vi "Gripper Controller.vi"(8 "error in":errorcluster) -> ()   [LabVIEW 2017]
doc: "This VI executes continuously carrying out the current operation and responding to updates or new operations. It will often contain the timing or control code that is difficult to place directly in TeleOp. This VI generally opens all sensors and motors and isolates the rest of the robot code from knowing how the operations are carried out."
uses:
  <vilib>/Rock Robotics/WPI/Framework/Completion Status.ctl
  Gripper Setpoints.ctl
  Gripper Operations.ctl
  <vilib>/Rock Robotics/SystemInterfaces/DIO/FPGA_DIOPWMChannel.ctl
  <vilib>/Rock Robotics/WPI/Solenoid/WPI_SolenoidChannel.ctl
  <vilib>/Rock Robotics/WPI/Solenoid/WPI_SolenoidValue.ctl
  <vilib>/Rock Robotics/WPI/MotorControl/WPI_MotorControlOpen SPARK.vi
  <vilib>/Rock Robotics/WPI/Solenoid/WPI_SolenoidOpenDouble.vi
  <vilib>/Rock Robotics/WPI/Solenoid/WPI_SolenoidSetEnum.vi
  <vilib>/addons/control/pid/pid.llb/PID Output Rate Limiter (DBL).vi
  <vilib>/Rock Robotics/SystemInterfaces/AI/FPGA_AIChannel.ctl
  <vilib>/addons/control/pid/NI_PID_pid.lvlib
  <vilib>/ptbypt/NI_PtbyPt.lvlib
panel:
  out "Peak":dbl
  in  "Speed Diff":dbl=0.8 format="%#_13g"
  in  "Peak Current":dbl=80.0
  in  "filter length":i32=50
  in  "output rate":dbl=1000.0 format="%.2f"
  out "Spinning?":bool
  out "Gripper":string
  out "Intake":string
  out "Currents":T1(graph)
  in  "Interactive Values":T2
  out "Current\nCmd":string
  in  "Buttons":cluster{"Execute Cmd":bool, "Abort Cmd":bool}
  out "Command Timing":cluster{"Start Time (ms)":u32, "Iterations":i32}
  out "Status":T4
  # "Interactive Command: You may fill in the settings for a command\nand schedule it with the Execute button. You can observe and abort\nany command while fine tuning the code for the controller."
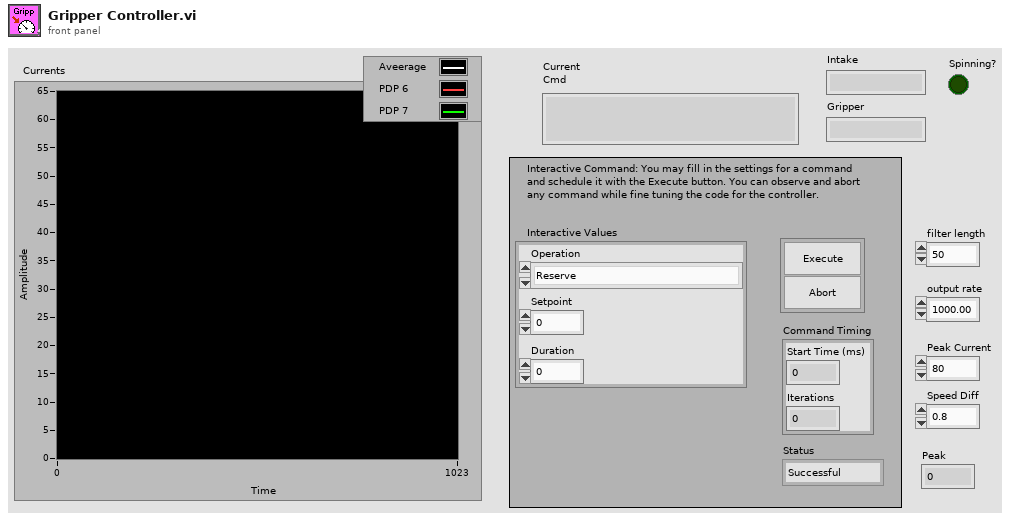
[diagram p1: front panel]
types:
  T1 = cluster{"mean":dbl, "Channel Current":dbl, "Channel Current":dbl}
  T2 = typedef "Gripper Setpoints.ctl" = cluster{"Operation":T3, "Setpoint":dbl, "Duration":dbl}
  T3 = typedef "Gripper Operations.ctl" = enum16{"Reserve", "Read Current", "Immediate", "Open", "Close", "Intake", "Shoot", "Stop"}
  T4 = typedef "Completion Status.ctl" = enum16{"Successful", "Aborted", "Incomplete"}
  T5 = typedef "WPI_SolenoidValue.ctl" = enum16{"Off", "On", "Forward", "Reverse"}
  T6 = typedef "WPI_SolenoidChannel.ctl" = enum8{"Solenoid 0", "Solenoid 1", "Solenoid 2", "Solenoid 3", "Solenoid 4", "Solenoid 5", "Solenoid 6", "Solenoid 7", "Invalid"}
  T7 = typedef "FPGA_DIOPWMChannel.ctl" = enum8{"PWM 0", "PWM 1", "PWM 2", "PWM 3", "PWM 4", "PWM 5", "PWM 6", "PWM 7", "PWM 8", "PWM 9", "PWM MXP 0", "PWM MXP 1", "PWM MXP 2", "PWM MXP 3", "PWM MXP 4", "PWM MXP 5", "PWM MXP 6", "PWM MXP 7", "PWM MXP 8", "PWM MXP 9", "Invalid"}
  T8 = typedef "WPI_SolenoidDevRef.ctl" = cluster{"DevStatus":errorcluster, "Pneumatics Control Module":u8, "Forward Solenoid Channel":T6, "Reverse Solenoid Channel":T6}
  T9 = typedef "WPI_MotorControlDeviceRef.ctl" = cluster{"DeviceStatus":errorcluster, "Type":T10, "PWM":cluster{"PWM Channel":T7, "DeadBand":T11}, "CAN":cluster{"Device Number":u8, "SetOutput VI Ref":variant, "GetOutput VI Ref":variant, "Enable VI Ref":variant, "Disable VI Ref":variant, "Data":variant}, "Invert":bool, "DIO PWM":cluster{"PWM \"Enable\" Channel":T7, "DIOChannel":T12, "PWM Rate":dbl}}
  T10 = typedef "WPI_MotorControlType.ctl" = enum16{"PWM", "CAN", "DIO PWM"}
  T11 = typedef "WPI_PWMDeadband.ctl" = cluster{"Name":string, "maxPositivePwm":i32, "minPositivePwm":i32, "centerPwm":i32, "maxNegativePwm":i32, "minNegativePwm":i32, "angularRange":u16}
  T12 = typedef "FPGA_DIOChannel.ctl" = enum8{"DIO 0", "DIO 1", "DIO 2", "DIO 3", "DIO 4", "DIO 5", "DIO 6", "DIO 7", "DIO 8", "DIO 9", "DIO MXP 0", "DIO MXP 1", "DIO MXP 2", "DIO MXP 3", "DIO MXP 4", "DIO MXP 5", "DIO MXP 6", "DIO MXP 7", "DIO MXP 8", "DIO MXP 9", "DIO MXP 10", "DIO MXP 11", "DIO MXP 12", "DIO MXP 13", "DIO MXP 14", "DIO MXP 15", "SPI Port CS1", "SPI Port CS2", "SPI Port CS3", "SPI Port MISO", "SPI Port MOSI", "Invalid"}
  T13 = typedef "FPGA_AIChannel.ctl" = enum8{"AI 0", "AI 1", "AI 2", "AI 3", "AI MXP 0", "AI MXP 1", "AI MXP 2", "AI MXP 3", "Invalid"}
  T14 = typedef "WPI_AnalogChannelDevRef.ctl" = cluster{"DevStatus":errorcluster, "Analog Channel":T13}
  T15 = typedef "Command Status Info.ctl" = cluster{"Name":string, "Status":T4, "notifier out":T16}
  T16 = typedef "Completion Notifier.ctl" = refnum<notifier>
  T17 = cluster{"Current Command":T2, "Command Timing":cluster{"Start Time (ms)":u32, "Iterations":i32}, "Command Arguments":cluster{"Command Info":T15, "Description":string, "Default Command":T2, "queue out":refnum<queue>, "Subsystem Name":string}}
  T18 = cluster{"MotorControlDevRef":T9, "MotorControlDevRef":T9, "SolenoidDevRef":T8}
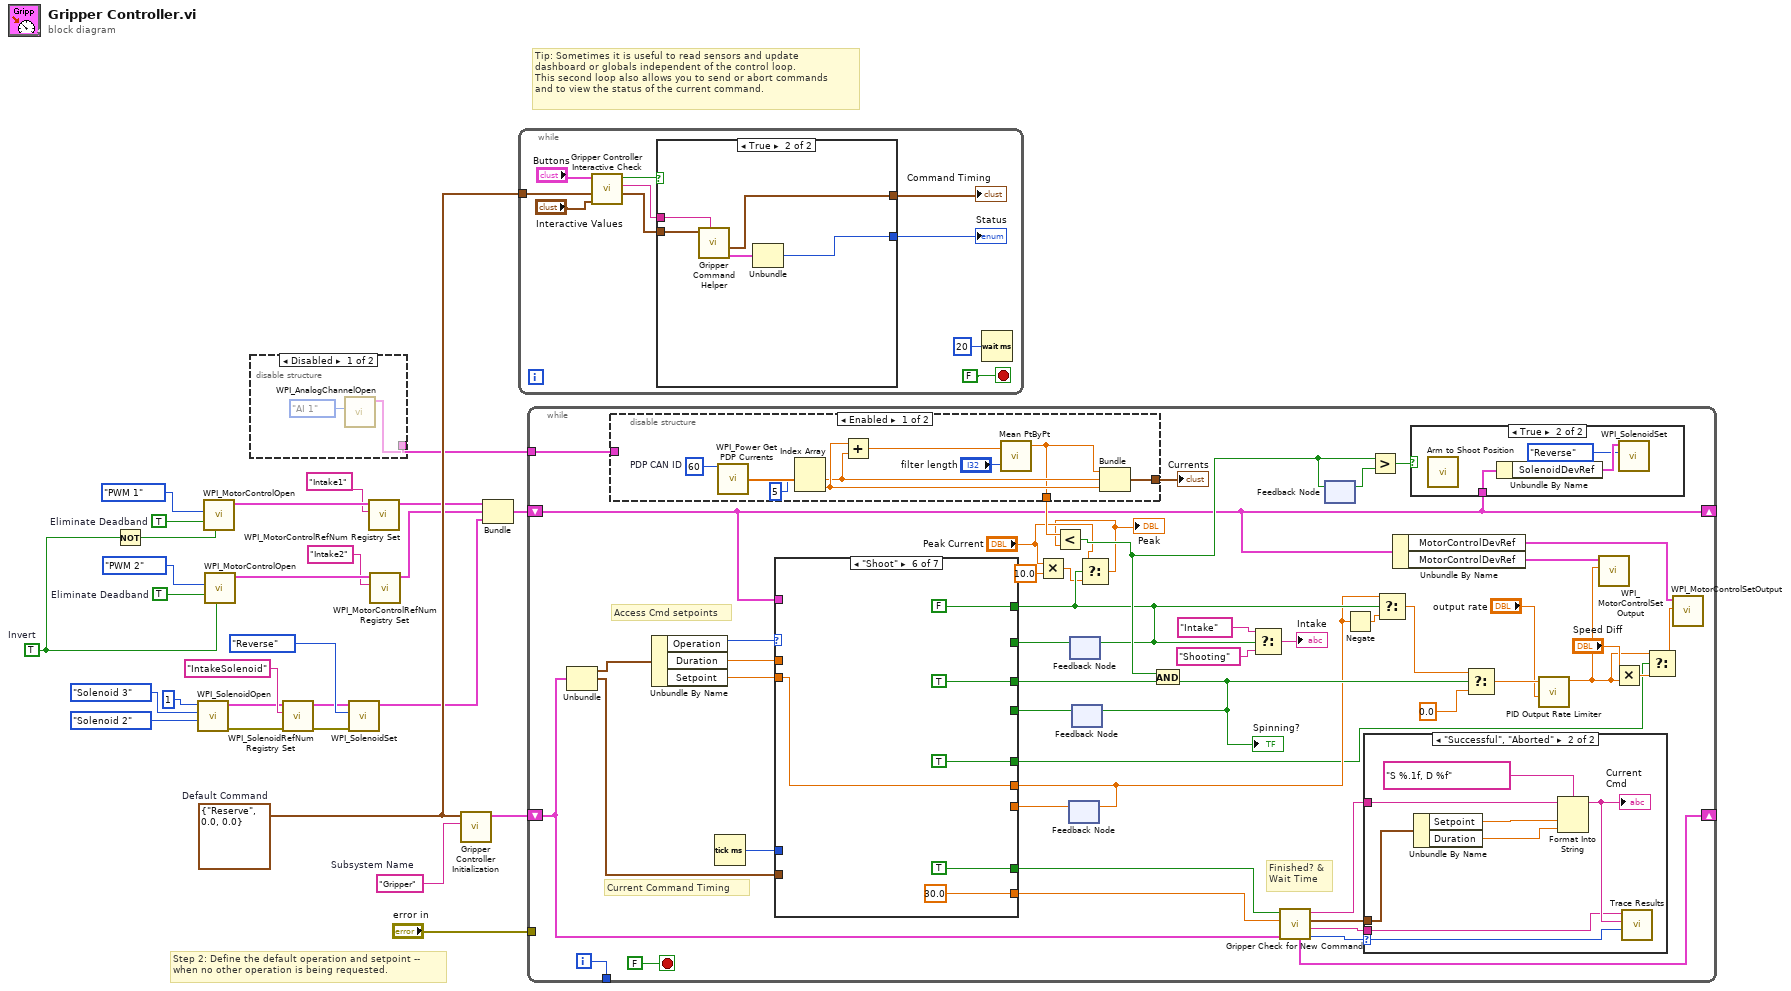
[diagram p0: block diagram]
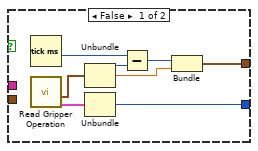
[diagram p3: hidden frame]
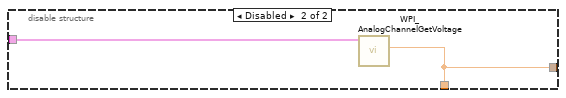
[diagram p4: hidden frame]
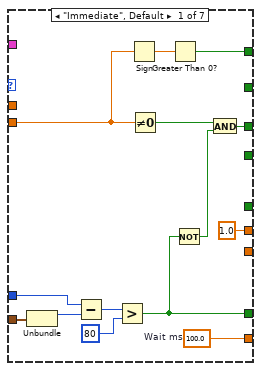
[diagram p7: hidden frame]
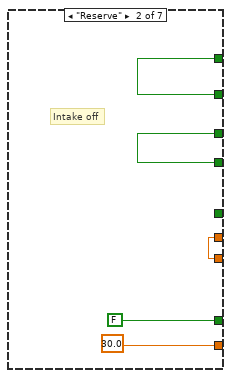
[diagram p8: hidden frame]
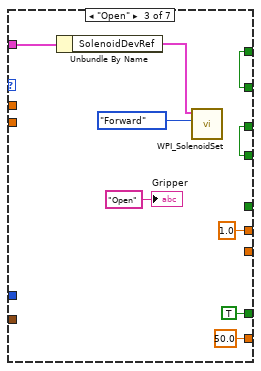
[diagram p9: hidden frame]
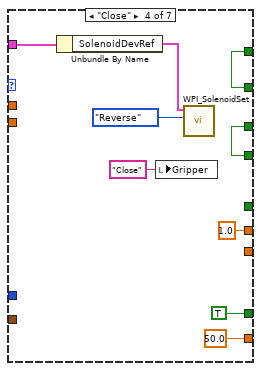
[diagram p10: hidden frame]
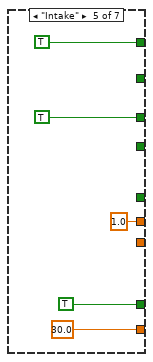
[diagram p11: hidden frame]
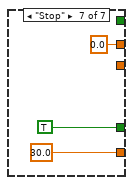
[diagram p12: hidden frame]
diagram:
  w24 = TRUE  # Invert
  w22 = TRUE  # Eliminate Deadband
  w18 = TRUE  # Eliminate Deadband
  w25 = T2 {"Operation"=enum."Reserve", "Setpoint"=0.0, "Duration"=0.0}  # Default Command
  w26 = "Gripper"  # Subsystem Name
  # "Tip: Sometimes it is useful to read sensors and update\ndashboard or globals independent of the control loop.\nThis second loop also allows you to send or abort commands\nand to view the status of the current command."
  # "Step 2: Define the default operation and setpoint --\nwhen no other operation is being requested."
  n1 = Not(x=w24) -> (.not. x?=w1:bool)
  n2 = call-poly <vilib>:"WPI_SolenoidOpen.vi"("Reverse Solenoid Channel"=WPI_SolenoidChannel."Solenoid 2", "Forward Solenoid Channel"=WPI_SolenoidChannel."Solenoid 3", "Pneumatics Control Module (0)"=u8 1) -> ("error out"=w9:errorcluster, "SolenoidDevRef"=w8:T8)  [unwired: 7 in]
  n3 = call-poly <vilib>:"WPI_MotorControlOpen.vi"("Invert"=w1, "Eliminate Deadband"=w18, "PWM Channel"=FPGA_DIOPWMChannel."PWM 1") -> ("MotorControlDeviceRef"=w19:T9)  [unwired: 7 in, 1 out]
  n4 = call-poly <vilib>:"WPI_MotorControlOpen.vi"("Invert"=w24, "Eliminate Deadband"=w22, "PWM Channel"=FPGA_DIOPWMChannel."PWM 2") -> ("MotorControlDeviceRef"=w21:T9)  [unwired: 7 in, 1 out]
  n5 = disable-structure shown="Disabled" {
    disable-tunnel: [w29 _] -> w2
    frame Disabled {
      n6 = call <vilib>:"WPI_AnalogChannelOpen.vi"("Analog Channel"=FPGA_AIChannel."AI 1") -> ("AIDeviceRef"=w29:T14)  [unwired: 9 in, 1 out]
    }
    frame Enabled {
    }
  }
  n7 = call <vilib>:"WPI_SolenoidRefNum Registry Set.vi"("error in (no error)"=w9, "refnum name"="IntakeSolenoid", "SolenoidDevRef"=w8) -> ("error out"=w12:errorcluster, "SolenoidDevRef"=w11:T8)  [unwired: 7 in]
  n8 = call-poly <vilib>:"WPI_SolenoidSet.vi"("error in (no error)"=w12, "Value"=WPI_SolenoidValue."Reverse", "SolenoidDevRef"=w11) -> ("SolenoidDevRef"=w4:T8)  [unwired: 7 in, 1 out]
  n9 = call <vilib>:"WPI_MotorControlRefNum Registry Set.vi"("refnum name"="Intake1", "MotorControlDevRef"=w19) -> ("MotorControlDevRef"=w15:T9)  [unwired: 8 in, 1 out]
  n10 = call <vilib>:"WPI_MotorControlRefNum Registry Set.vi"("refnum name"="Intake2", "MotorControlDevRef"=w21) -> ("MotorControlDevRef"=w14:T9)  [unwired: 8 in, 1 out]
  n11 = call "Gripper Controller Initialization.vi"("Subsystem Name"=w26, "Default Command"=w25) -> ("Current Command"=w27:T17)  [unwired: 9 in]
  n12 = Bundle("MotorControlDevRef"=w15, "MotorControlDevRef"=w14, "SolenoidDevRef"=w4) -> (w3:T18)  [unwired: 1 in]
  n13 = while {
    tunnel: w25 -> [w37]
    stop <- FALSE stop-if-true
    n14 = call "Gripper Controller Interactive Check.vi"("Interactive Command in"="Interactive Values", "Default Command"=w37, "Buttons"="Buttons") -> ("Interactive Command out"=w34:T2, "Trace String"=w35:string, "Schedule"=w36:bool)  [unwired: 6 in]
    n15 = case shown="True" w36 {
      tunnel: [w48 w53] -> w33
      tunnel: w34 -> [_ w51]
      tunnel: [w44 w49] -> w32
      tunnel: w35 -> [_ w52]
      frame False {
        n16 = Tick Count (ms)() -> (millisecond timer value=w43:u32)
        n17 = call "Read Gripper Operation.vi"() -> ("Command Info"=w41:T15, "SubSystem Data"=w42:T2)  [unwired: 9 in, 1 out]
        n18 = Unbundle(w42) -> ("Operation"=w47:T3, "Setpoint"=w45:dbl)  [unwired: 1 out]
        n19 = Unbundle(w41) -> ("Status"=w48:T4)  [unwired: 2 out]
        n20 = Subtract(x=w43, y=w47) -> (x-y=w46:u32)
        n21 = Bundle(w46, "Setpoint"=w45) -> (w44:cluster{u32, "Setpoint":dbl})  [unwired: 1 in]
      }
      frame True {
        n22 = call "Gripper Command Helper.vi"("Description"=w52, "SubSystem Data"=w51) -> ("Command Info Out"=w50:T15, "Command Timing"=w49:cluster{"Start Time (ms)":u32, "Iterations":i32})  [unwired: 7 in, 1 out]
        n23 = Unbundle(w50) -> ("Status"=w53:T4)  [unwired: 2 out]
      }
    }
    "Status" <- w33
    "Command Timing" <- w32
    n24 = Wait (ms)(milliseconds to wait=u32 20) -> ()  [unwired: 1 out]
  }
  n25 = while {
    shift-right: [w94] -> _
    shift-left: w27 -> [w87]
    tunnel: [w101] -> _
    tunnel: "error in" -> [_]
    shift-right: [w67] -> _
    shift-left: w3 -> [w67]
    tunnel: w2 -> [w66]
    i -> [w101]
    stop <- FALSE stop-if-true
    # "Current Command Timing"
    # "Access Cmd setpoints"
    # "Finished? &\nWait Time"
    n26 = Unbundle(w87) -> ("Current Command"=w100:T2, "Command Timing"=w96:cluster{"Start Time (ms)":u32, "Iterations":i32})  [unwired: 1 out]
    n27 = disable-structure shown="Enabled" {
      disable-tunnel: [w109 w112] -> w75
      disable-tunnel: [w103 w112] -> w72
      disable-tunnel: w66 -> [_ w113]
      frame Enabled {
        w111 = u8 60  # PDP CAN ID
        n28 = call <vilib>:"WPI_Power Get PDP Currents.vi"("Power Distribution Panel (0)"=w111) -> ("all currents (A)"=w110:dbl[])  [unwired: 12 in, 2 out]
        n29 = Index Array(array=w110, index #1=5 ("index")) -> (element #1=w106:dbl, element #2=w107:dbl)  [unwired: 1 in]
        n30 = Add(x=w107, y=w106) -> (x+y=w105:dbl)
        n31 = call <vilib>:"Mean PtByPt.vi"("x"=w105, "sample length"="filter length") -> ("mean"=w103:dbl)  [unwired: 2 in, 1 out]
        n32 = Bundle("mean"=w103, "Channel Current"=w106, "Channel Current"=w107) -> (w109:T1)  [unwired: 1 in]
      }
      frame Disabled {
        n33 = call <vilib>:"WPI_AnalogChannelGetVoltage.vi"("AIDeviceRef"=w113) -> ("Voltage"=w112:dbl)  [unwired: 8 in, 2 out]
      }
    }
    "Currents" <- w75
    n34 = Unbundle By Name(w100) -> ("Operation"=w99:T3, "Duration"=w98:dbl, "Setpoint"=w95:dbl)
    n35 = Tick Count (ms)() -> (millisecond timer value=w97:u32)
    n36 = Multiply(x="Peak Current", y=10.0) -> (x*y=w61:dbl)
    n37 = feedback #1() -> (w58:dbl)  [unwired: 1 in]
    n38 = feedback #2() -> (w81:bool)  [unwired: 1 in]
    n39 = feedback #3() -> (w80:bool)  [unwired: 1 in]
    n40 = case shown="\"Shoot\"" w99 {
      tunnel: [w138 30.0 50.0 ("Infinite") 50.0 ("Infinite") 30.0 ("Infinite") 30.0 ("Infinite") 30.0 ("Infinite")] -> w92
      tunnel: [w127 FALSE ("ignore previous (F)") TRUE ("ignore previous (F)") TRUE ("ignore previous (F)") TRUE ("ignore previous (F)") TRUE ("ignore previous (F)") TRUE ("ignore previous (F)")] -> w93
      tunnel: w96 -> [w134 _ _ _ _ _ _]
      tunnel: w98 -> [_ _ _ _ _ _ _]
      tunnel: w97 -> [w133 _ _ _ _ _ _]
      tunnel: w95 -> [w130 _ _ _ _ w168 _]
      tunnel: w67 -> [_ _ w152 w161 _ _ _]
      tunnel: [w128 w140 w146 w155 TRUE TRUE _] -> w79
      tunnel: [w131 w141 w147 w156 TRUE FALSE _] -> w63
      tunnel: w81 -> [_ w141 w147 w156 _ _ _]
      tunnel: w80 -> [_ w140 w146 w155 _ _ _]
      tunnel: [1.0 ("Setpoint") w139 1.0 ("Setpoint") 1.0 ("Setpoint") 1.0 ("Setpoint") w168 0.0 ("Setpoint")] -> w59
      tunnel: w58 -> [_ w139 _ _ _ _ _]
      tunnel: [_ _ _ _ _ TRUE _] -> w54
      frame "Immediate", Default {
        w138 = 100.0  # Wait ms
        n41 = Unbundle(w134) -> ("Start Time (ms)"=w137:u32)  [unwired: 1 out]
        n42 = Subtract(x=w133, y=w137) -> (x-y=w136:u32)
        n43 = Greater?(x=w136, y=u8 80 ("Left Motor")) -> (0:w127:bool)
        n44 = Sign(1:w130) -> (0:w132:dbl)
        n45 = Not Equal To 0?(x=w130) -> (x != 0?=w129:bool)
        n46 = Greater Than 0?(x=w132) -> (x > 0?=w131:bool)
        n47 = Not(x=w127) -> (.not. x?=w126:bool)
        n48 = And(x=w129, y=w126) -> (x .and. y?=w128:bool)
      }
      frame "Reserve" {
        # "Intake off"
      }
      frame "Open" {
        n49 = Unbundle By Name(w152) -> ("SolenoidDevRef"=w151:T8)
        n50 = call-poly <vilib>:"WPI_SolenoidSet.vi"("Value"=WPI_SolenoidValue."Forward", "SolenoidDevRef"=w151) -> ()  [unwired: 8 in, 2 out]
        "Gripper" <- "Open" ("Gripper")
      }
      frame "Close" {
        n51 = Unbundle By Name(w161) -> ("SolenoidDevRef"=w160:T8)
        n52 = local write "Gripper"("Close" ("Gripper")) -> ()
        n53 = call-poly <vilib>:"WPI_SolenoidSet.vi"("Value"=WPI_SolenoidValue."Reverse", "SolenoidDevRef"=w160) -> ()  [unwired: 8 in, 2 out]
      }
      frame "Intake" {
      }
      frame "Shoot" {
      }
      frame "Stop" {
      }
    }
    n54 = feedback-in #1(w59) -> ()
    n55 = feedback-in #2(w63) -> ()
    n56 = Select(t="Peak Current", s=w63, f=w61) -> (s? t:f=w60:dbl)
    "Peak" <- w60
    n57 = Less?(x=w72, y=w60) -> (x < y?=w68:bool)
    n58 = And(x=w68, y=w79) -> (x .and. y?=w71:bool)
    "Spinning?" <- w71
    n59 = feedback-in #3(w71) -> ()
    n60 = Select(t="Intake" ("format string"), s=w63, f="Shooting" ("format string")) -> (s? t:f=→"Intake":string)
    n61 = call "Gripper Check for New Command.vi"("Current Command"=w87, "Wait time (ms)"=w92, "Finished?"=w93) -> ("Completion"=w88:T4, "Subsystem Name"=w89:string, "Current Command"=w90:T2, "Initial Trace String"=w91:string, "NextCommand"=w94:T17)  [unwired: 4 in]
    n62 = feedback-in #4(w68) -> ()
    n63 = feedback #4() -> (w70:bool)  [unwired: 1 in]
    n64 = Negate(x=w59) -> (-x=w82:dbl)
    n65 = case shown="\"Successful\", \"Aborted\"" w88 {
      selector: w88 -> [_ w124]
      tunnel: w91 -> [_ w120]
      tunnel: w90 -> [_ w121]
      tunnel: w89 -> [_ w117]
      frame "Incomplete", Default {
        # "Continuing current command"
      }
      frame "Successful", "Aborted" {
        # "Report and setup for next command"
        n66 = Unbundle By Name(w121) -> ("Setpoint"=w123:dbl, "Duration"=w118:dbl)
        n67 = Format Into String(format string="S %.1f, D %f", initial string=w120, w123, w118) -> (resulting string=w119:string)  [unwired: 1 in, 1 out]
        "Current\nCmd" <- w119
        n68 = call <vilib>:"Trace Results.vi"("Status of previous command"=w124, "Description"=w119, "Subsystem"=w117) -> ()  [unwired: 9 in]
      }
    }
    n69 = Greater?(x=w68, y=w70) -> (0:w69:bool)
    n70 = Select(t=w59, s=w63, f=w82) -> (s? t:f=w83:dbl)
    n71 = Unbundle By Name(w67) -> ("MotorControlDevRef"=w85:T9, "MotorControlDevRef"=w86:T9)
    n72 = case shown="True" w69 {
      tunnel: w67 -> [_ w114]
      frame False {
      }
      frame True {
        n73 = call "Arm to Shoot Position.vi"() -> ()  [unwired: 11 in, 1 out]
        n74 = Unbundle By Name(w114) -> ("SolenoidDevRef"=w116:T8)
        n75 = call-poly <vilib>:"WPI_SolenoidSet.vi"("Value"=WPI_SolenoidValue."Reverse", "SolenoidDevRef"=w116) -> ()  [unwired: 8 in, 2 out]
      }
    }
    n76 = Select(t=w83, s=w71, f=0.0) -> (s? t:f=w74:dbl)
    n77 = call-poly <vilib>:"PID Output Rate Limiter.vi"("output rate (EGU/min)"="output rate", "input (controller output)"=w74) -> ("output"=w55:dbl)  [unwired: 6 in, 1 out]
    n78 = call <vilib>:"WPI_MotorControlSetOutput.vi"("Output"=w55, "MotorControlDevRef"=w86) -> ()  [unwired: 7 in, 3 out]
    n79 = Multiply(x="Speed Diff", y=w55) -> (x*y=w56:dbl)
    n80 = Select(t=w55, s=w54, f=w56) -> (s? t:f=w57:dbl)
    n81 = call <vilib>:"WPI_MotorControlSetOutput.vi"("Output"=w57, "MotorControlDevRef"=w85) -> ()  [unwired: 7 in, 3 out]
  }
